vi "PV ActiveLine - CalibrationFactor (TPG362).vi"(7 "W/R":bool, 8 "Fehler (Eingang)":errorcluster, 9 "Set Calibration factor2":dbl=1.0 min=0.1 max=9.999 step=0.001 format="%.3f", 10 "Set Calibration factor1":dbl=1.0 min=0.1 max=9.999 step=0.001 format="%.3f", 11 "Referenz in":refnum<visa-resource-name>) -> (0 "Cluster (Ausgang)":errorcluster, 1 "Get Calibration factor 2":dbl=0.000753 format="%.3f", 2 "Get Calibration factor 1":dbl=0.000753 format="%.3f", 3 "Referenz out":refnum<visa-resource-name>)   [LabVIEW 2013, in "PV ActiveLine.lvlib"]
doc: "COR - Correction Factor\n\nCOR corresponds to the CAL command\n\nTransmit: COR [,a.aaa,b.bbb]\nReceive: a.aaa,b.bbb\n\na.aaa = Correction factor gauge 1\nb.bbb = Correction factor gauge 2"
uses:
  C:/Program Files (x86)/National Instruments/LabVIEW 2013/PV ActiveLine/PV ActiveLine.lvlib
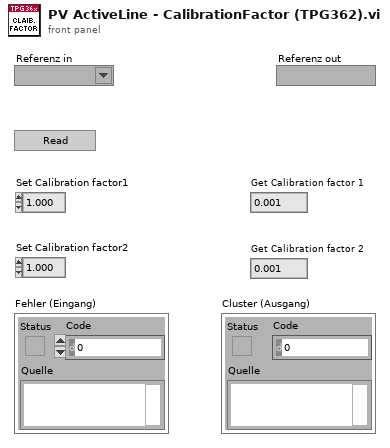
[diagram p1: front panel]
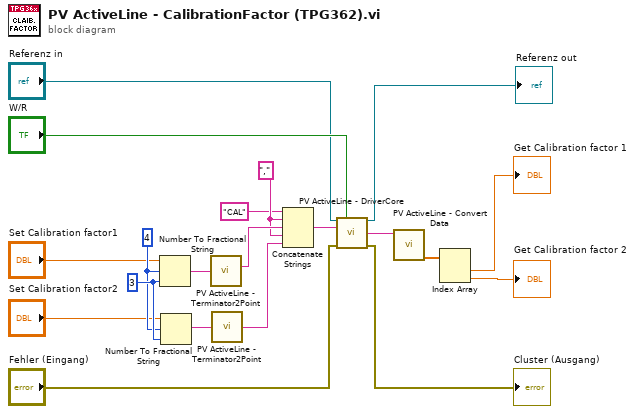
[diagram p0: block diagram]
diagram:
  w7 = i16 4 ("width (-)")
  w8 = i16 3 ("width (-)")
  w6 = ","
  n1 = Number To Fractional String(number="Set Calibration factor1", width (-)=w7, precision (6)=w8) -> (F-format string=w11:string)  [unwired: 1 in]
  n2 = Number To Fractional String(number="Set Calibration factor2", width (-)=w7, precision (6)=w8) -> (F-format string=w10:string)  [unwired: 1 in]
  n3 = call "PV ActiveLine - Terminator2Point.vi"("Eingangstring"=w11) -> ("Ausgangstring"=w9:string)
  n4 = call "PV ActiveLine - Terminator2Point.vi"("Eingangstring"=w10) -> ("Ausgangstring"=w5:string)
  n5 = Concatenate Strings("CAL", w6, w9, w6, w5) -> (w4:string)
  n6 = call "PV ActiveLine - DriverCore.vi"("Referenz in"="Referenz in", "Write/Read"="W/R", "Command"=w4, "Fehler (Eingang)"="Fehler (Eingang)") -> ("Referenz out"=→"Referenz out":refnum<visa-resource-name>, "String Out"=w15:string, "Cluster (Ausgang)"=→"Cluster (Ausgang)":errorcluster)  [unwired: 9 in]
  n7 = call "PV ActiveLine - Convert Data.vi"("String in"=w15) -> ("DBL out"=w14:dbl[])  [unwired: 7 in, 3 out]
  n8 = Index Array(array=w14) -> (element #1=→"Get Calibration factor 1":dbl, element #2=→"Get Calibration factor 2":dbl)  [unwired: 2 in]
